vi "Obtain Message Queue.vi"(8 "error in (no error)":errorcluster, 11 "Queue name":string[](array[string])) -> (0 "error out":errorcluster, 3 "Message Queue":refnum<queue>)   [LabVIEW 2016, in "Message Queue.lvlib"]
doc: "Create array queue handler with the Message Cluster data type."
uses:
  Message Queue.lvlib
  Message Cluster.ctl
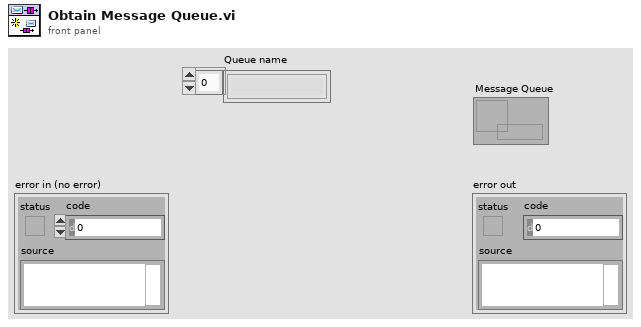
[diagram p1: front panel]
types:
  T1 = typedef "Message Queue.lvlib/Message Cluster.ctl" = cluster{"Message":string, "Message Data":variant}
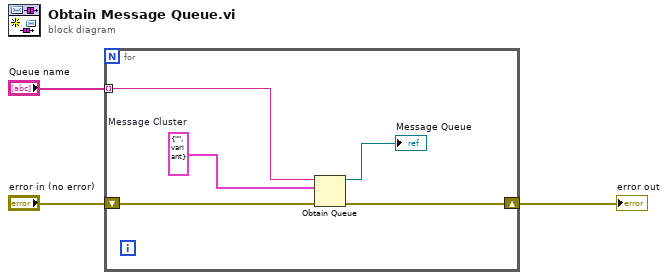
[diagram p0: block diagram]
diagram:
  n1 = for {
    shift-right: [w5] -> w2
    shift-left: "error in (no error)" -> [w7]
    tunnel: "Queue name" -> [w4] mode=indexing
    w8 = T1 {"Message"="", "Message Data"=variant}  # Message Cluster
    n2 = Obtain Queue(name (unnamed)=w4, element data type=w8, error in (no error)=w7) -> (queue out=→"Message Queue":refnum<queue>, error out=w5:errorcluster)  [unwired: 2 in, 1 out]
  }
  "error out" <- w2
